vi "Skidpad.vi"() -> ()   [LabVIEW 2020]
uses:
  Control/SkidpadBestRecordIndicator.ctl
  Control/SkidpadCurrentRecordIndicator.ctl
  Control/SkidpadInternalVariable.ctl
  CommonControl/Flag.ctl
  Control/SkidpadInternalTimmer.ctl
  Control/SkidpadState.ctl
  <vilib>/DAQmx/write.llb/DAQmx Write (Analog DBL 1Chan 1Samp).vi
  <vilib>/DAQmx/read.llb/DAQmx Read (Analog DBL 1Chan 1Samp).vi
  <vilib>/DAQmx/create/channels.llb/DAQmx Create Channel (AO-Voltage-Basic).vi
  <vilib>/DAQmx/create/channels.llb/DAQmx Create Channel (AI-Voltage-Basic).vi
  <vilib>/Utility/file.llb/Read Delimited Spreadsheet (string).vi
  <vilib>/DAQmx/miscellaneous.llb/DAQmx Fill In Error Info.vi
  <vilib>/Utility/file.llb/Write Delimited Spreadsheet (string).vi
panel:
  out "Progress":string[][](table)
  in  "DNF":bool
  in  "DeviceName":tag
  in  "NextEntry":bool
  in  "Ready":bool
  in  "Retry":bool
  out "CurrentRecordIndicator":T1
  out "BestRecordIndicator":T2
  in  "ProgramStop":bool
  # "2023 KSAE Formula Skidpad Event"
  # "Team"
  # "Entry"
  # "Hit"
  # "University"
  # "Lap2 :"
  # "Lap4 :"
  # "Total :"
  # "Entry :"
  # "#1"
  # "#2"
  # "#3"
  # "#4"
  # "Univ. :"
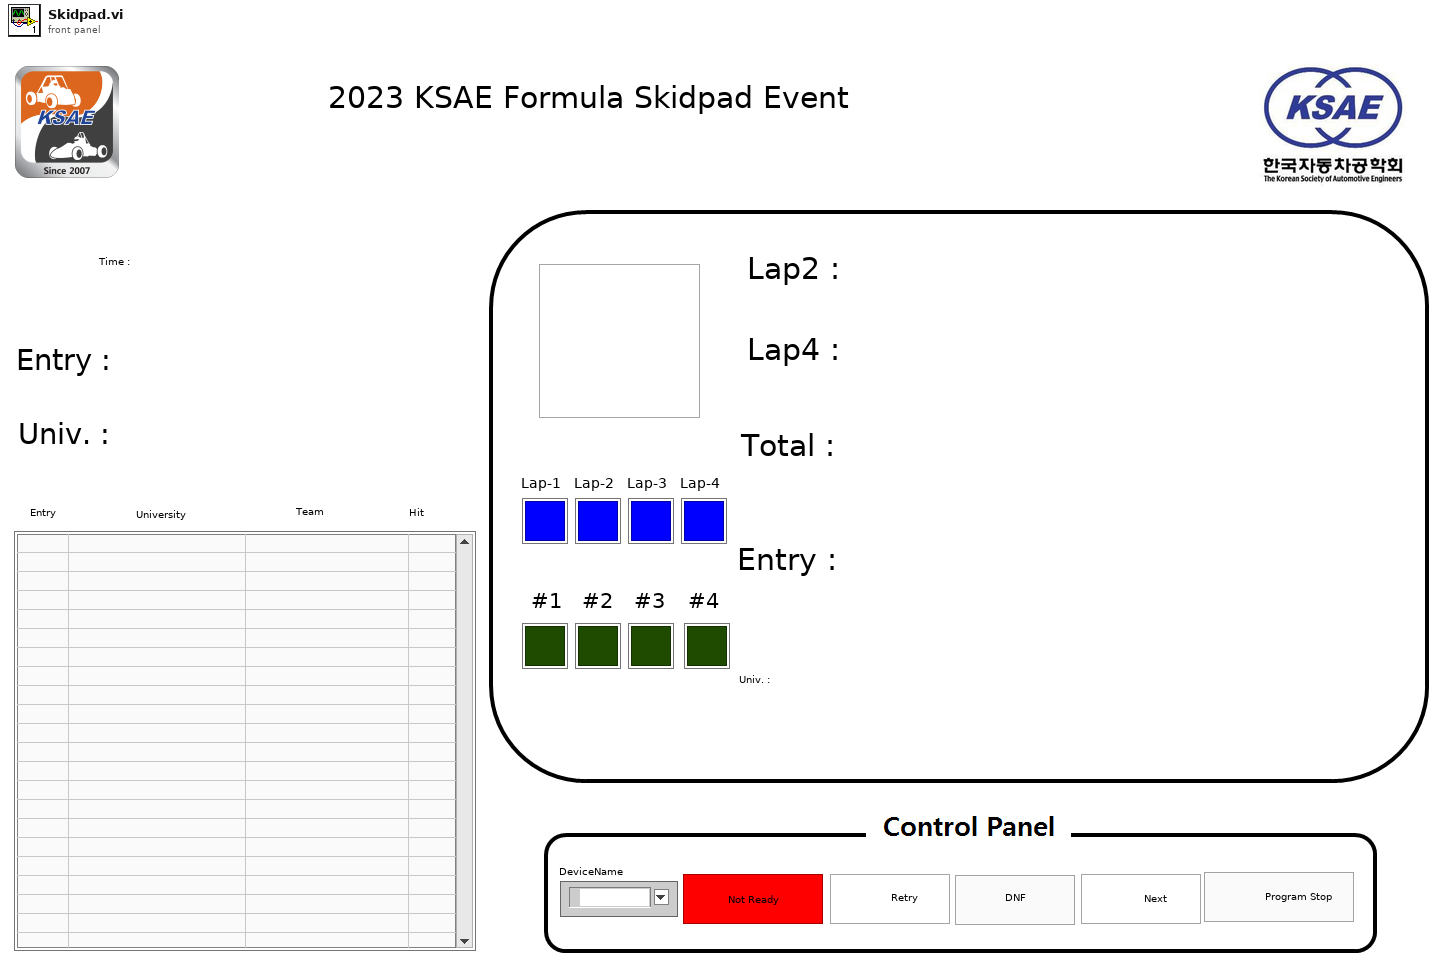
[diagram p1: front panel]
types:
  T1 = typedef "SkidpadCurrentRecordIndicator.ctl" = cluster{"Lab2":string, "Lab4":string, "TotalLabTime":string, "CurrentEntry":string, "CurrentSchool":string, "Flag":picture, "Message":string, "LapProgress":cluster{"Lap-1":bool, "Lap-2":bool, "Lap-3":bool, "Lap-4":bool}, "EventCount":cluster{"Attempt-1":bool, "Attempt-2":bool, "Attempt-3":bool, "Attempt-4":bool}}
  T2 = typedef "SkidpadBestRecordIndicator.ctl" = cluster{"BestTime":string, "BestEntry":string, "BestUniv":string}
  T3 = typedef "SkidpadInternalVariable.ctl" = cluster{"CurrentRecordIndicator":T1, "BestRecordIndicator":T2, "FlagData":T4, "InternalTimmer":T5, "StateValue":T6, "EventProgressData":string[][], "Ready":bool, "Retry":bool, "DNF":bool, "NextEntry":bool, "ProgramStop":bool}
  T4 = typedef "Flag.ctl" = cluster{"GreenFlag":picture, "BlueFlag":picture, "RedFlag":picture, "CheckFlag":picture}
  T5 = typedef "SkidpadInternalTimmer.ctl" = cluster{"1LapRefTime":i64, "1LapTime":i64, "2LapRefTime":i64, "2LapTime":i64, "3LapRefTime":i64, "3LapTime":i64, "4LapRefTime":i64, "4LapTime":i64, "TotalLabTime":i64}
  T6 = typedef "SkidpadState.ctl" = enum16{"Initial", "InputInfomation", "Ready", "1lap", "2lap", "3lap", "4lap", "FinshRunning", "LogRecord", "HardwareRelease", "WaittingforNext", "ProgramStop"}
  T7 = cluster{"Lap-1":bool, "Lap-2":bool, "Lap-3":bool, "Lap-4":bool}
  T8 = cluster{"CurrentEntry":string, "CurrentUniversity":string, "CurrentTeam":string}
  T9 = cluster{"Attempt-1":bool, "Attempt-2":bool, "Attempt-3":bool, "Attempt-4":bool}
  T10 = cluster{"Lab1":bool, "Lab2":bool, "Lab3":bool, "Lab4":bool}
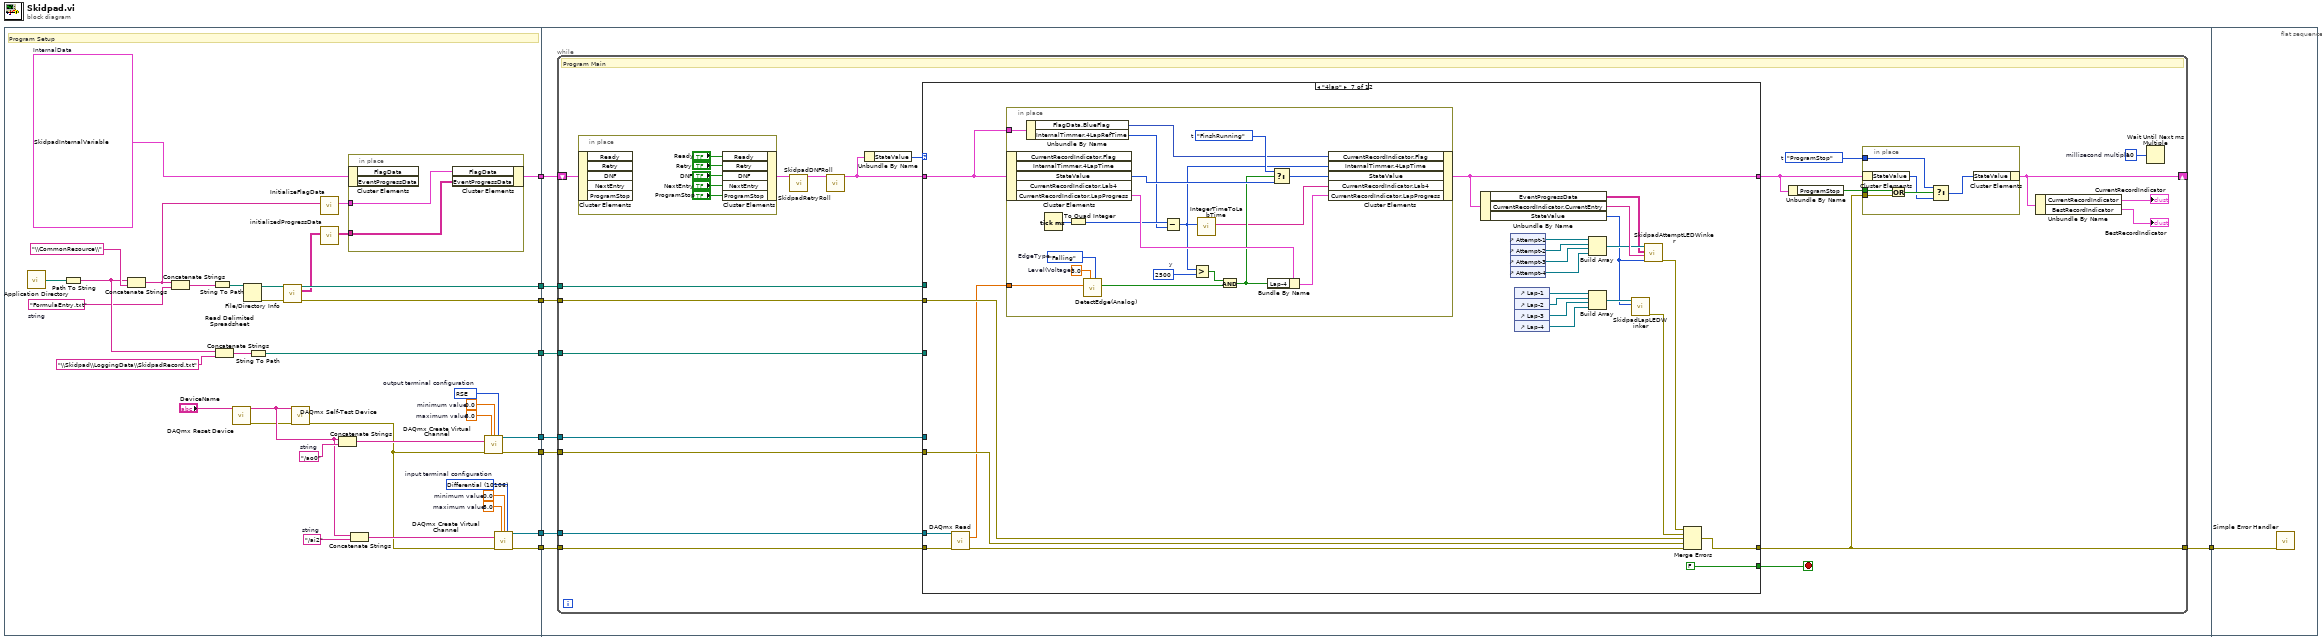
[diagram p0: block diagram]
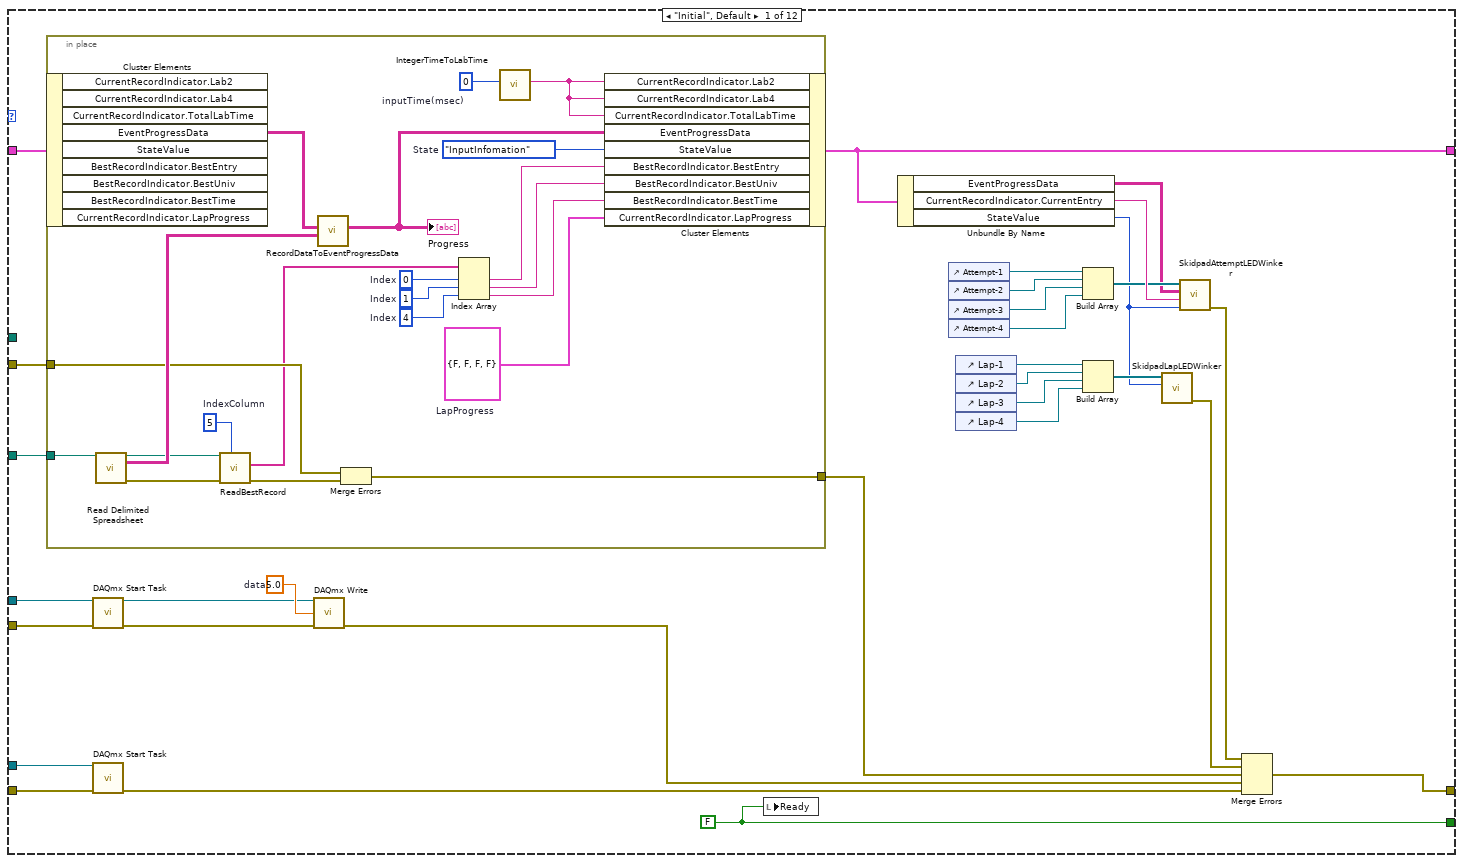
[diagram p2: hidden frame]
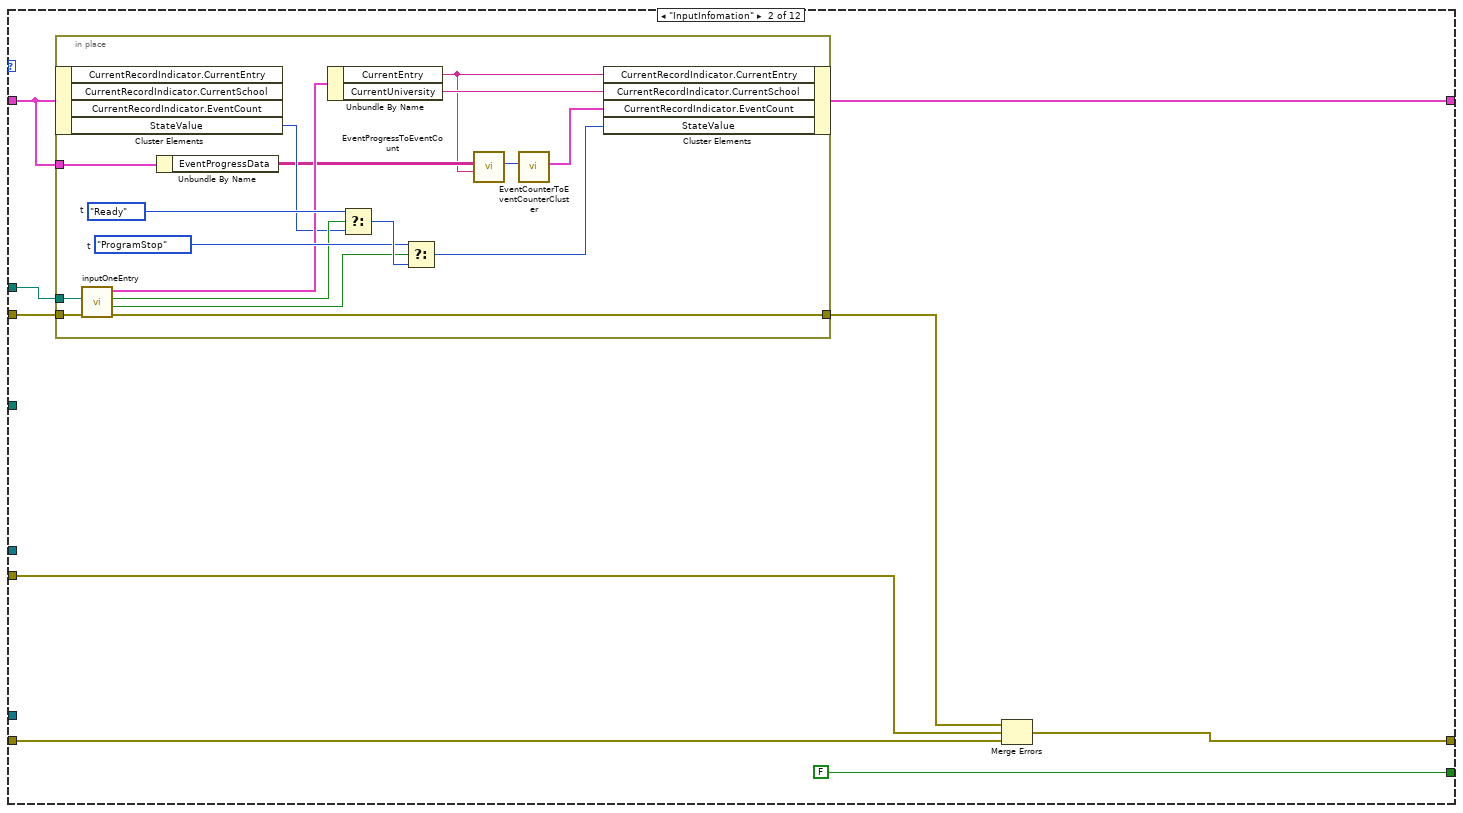
[diagram p3: hidden frame]
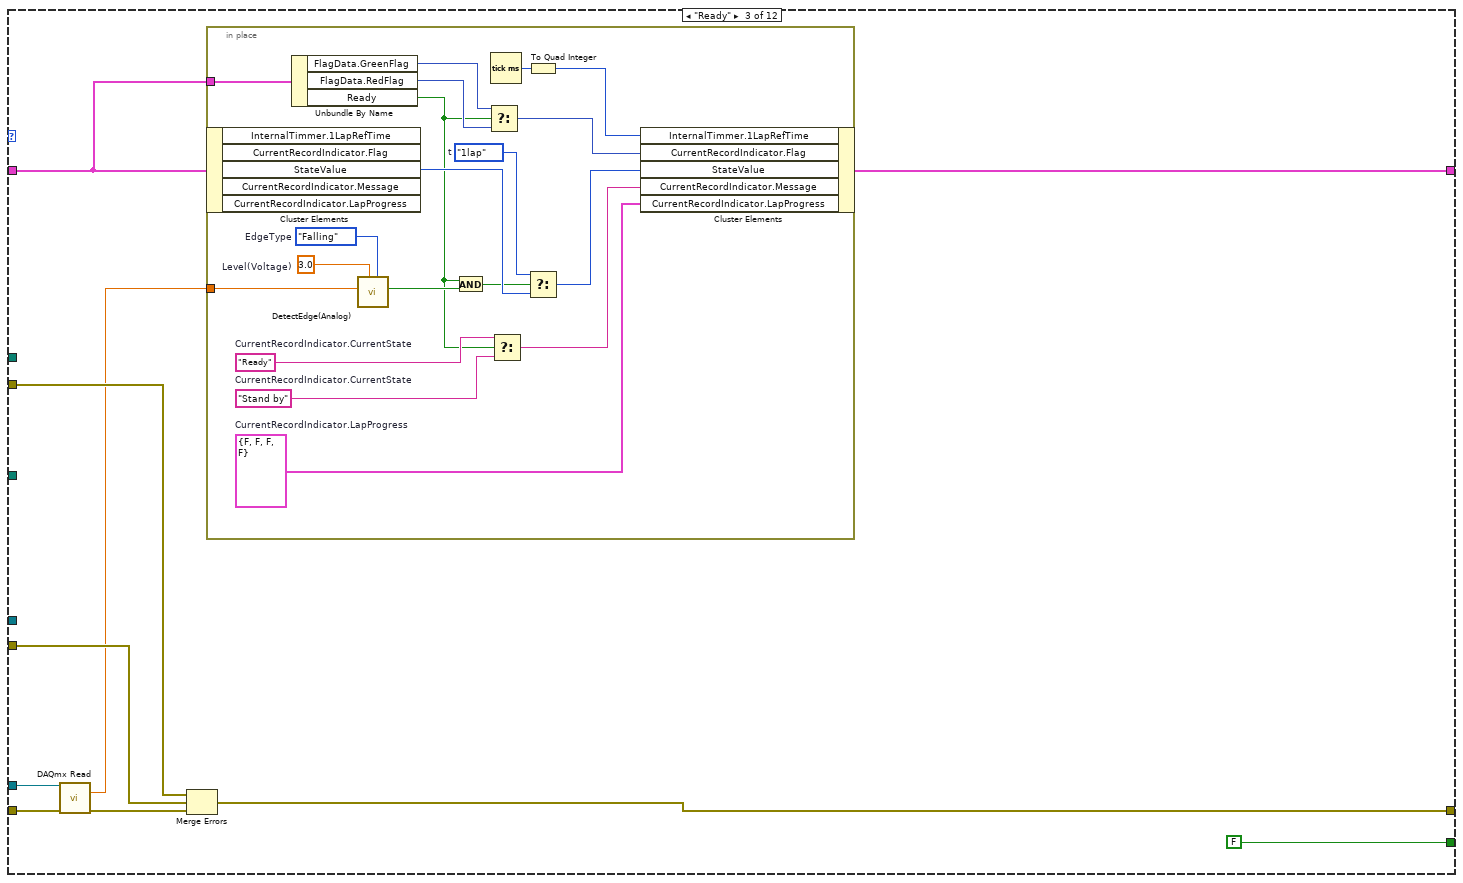
[diagram p4: hidden frame]
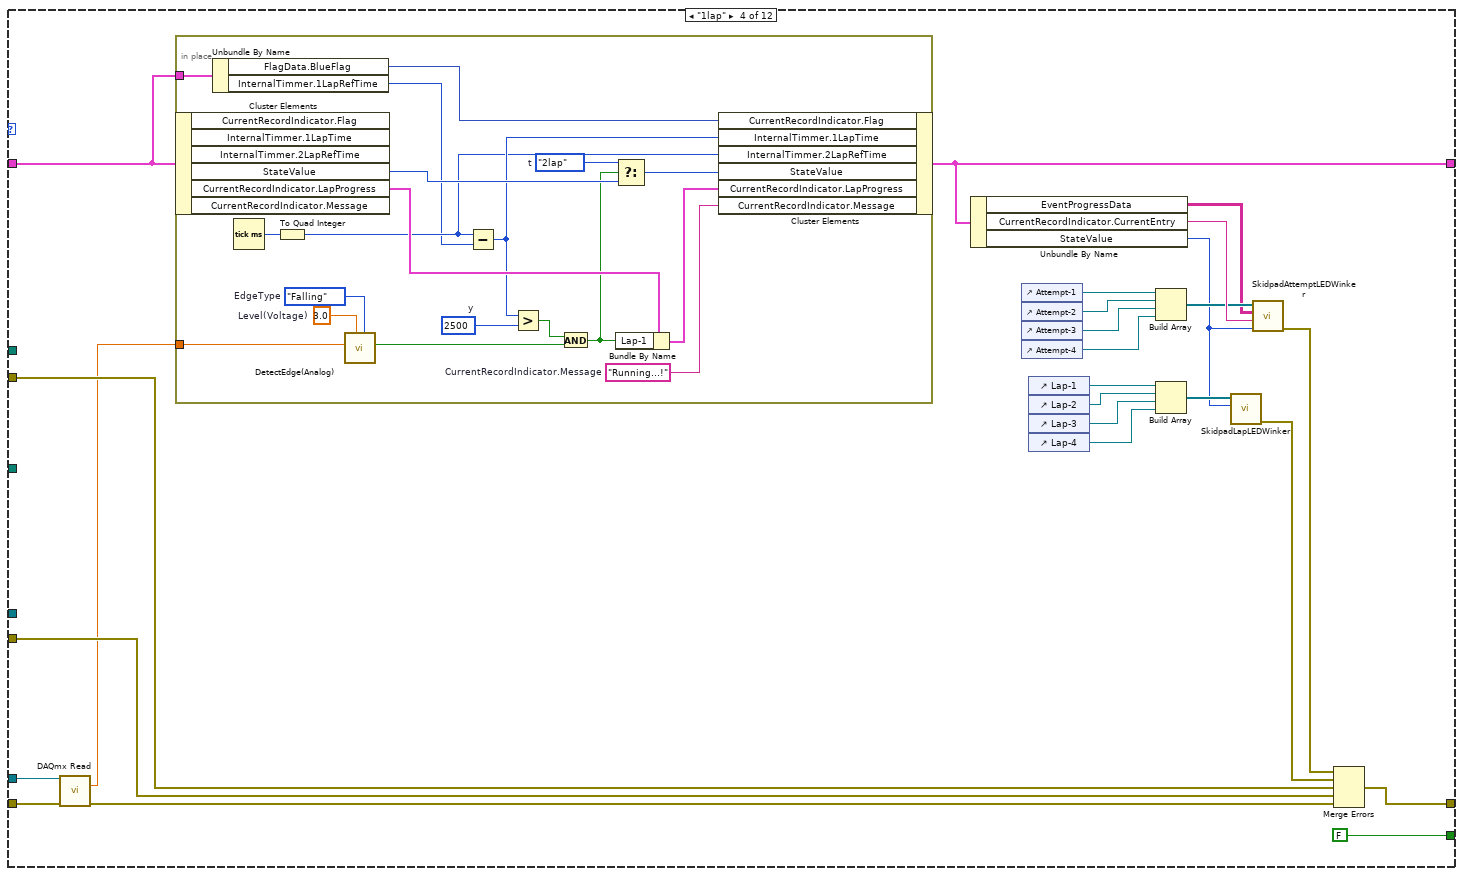
[diagram p5: hidden frame]
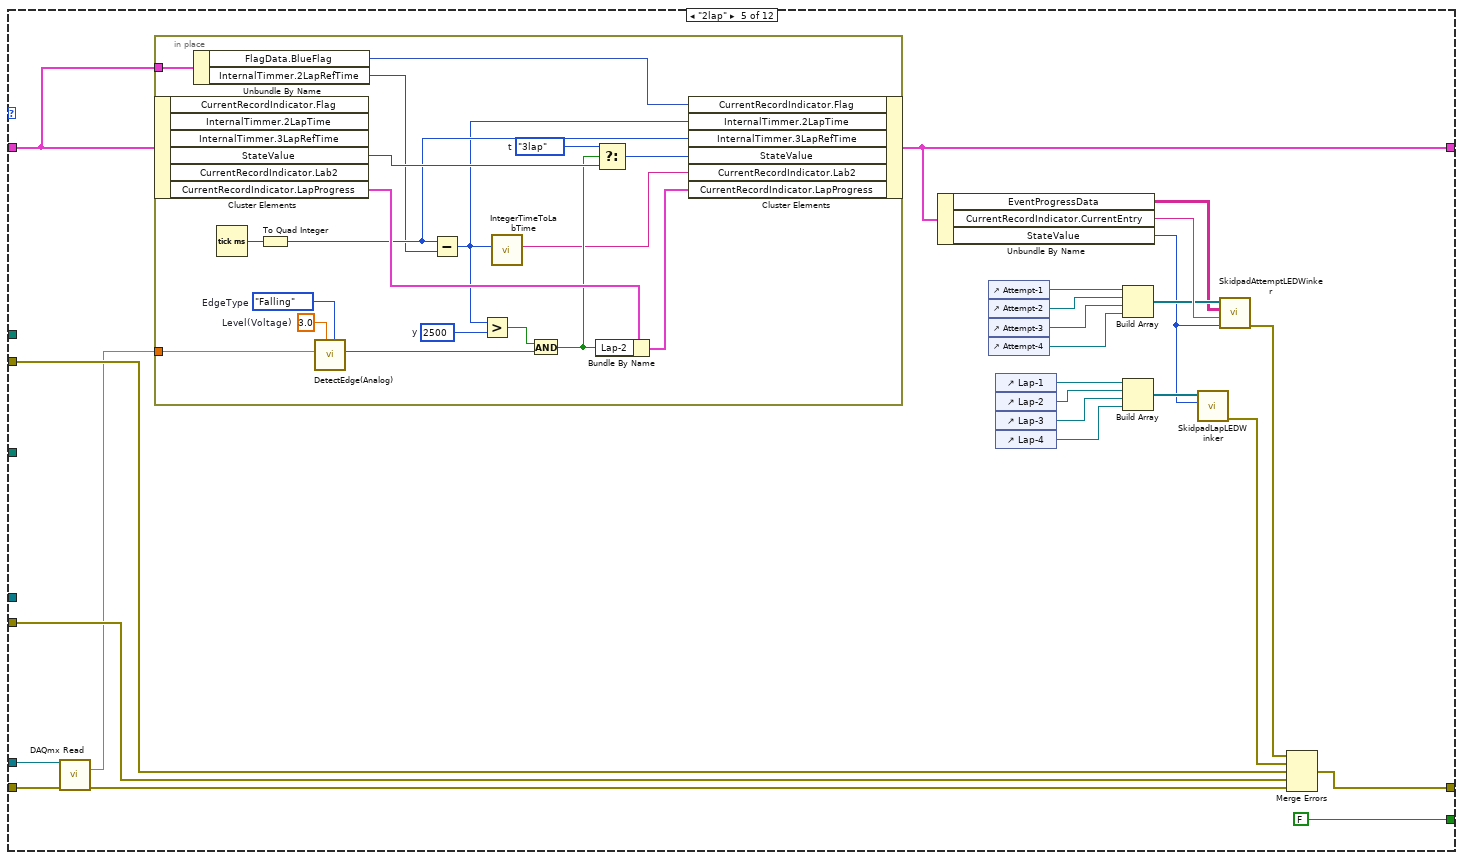
[diagram p6: hidden frame]
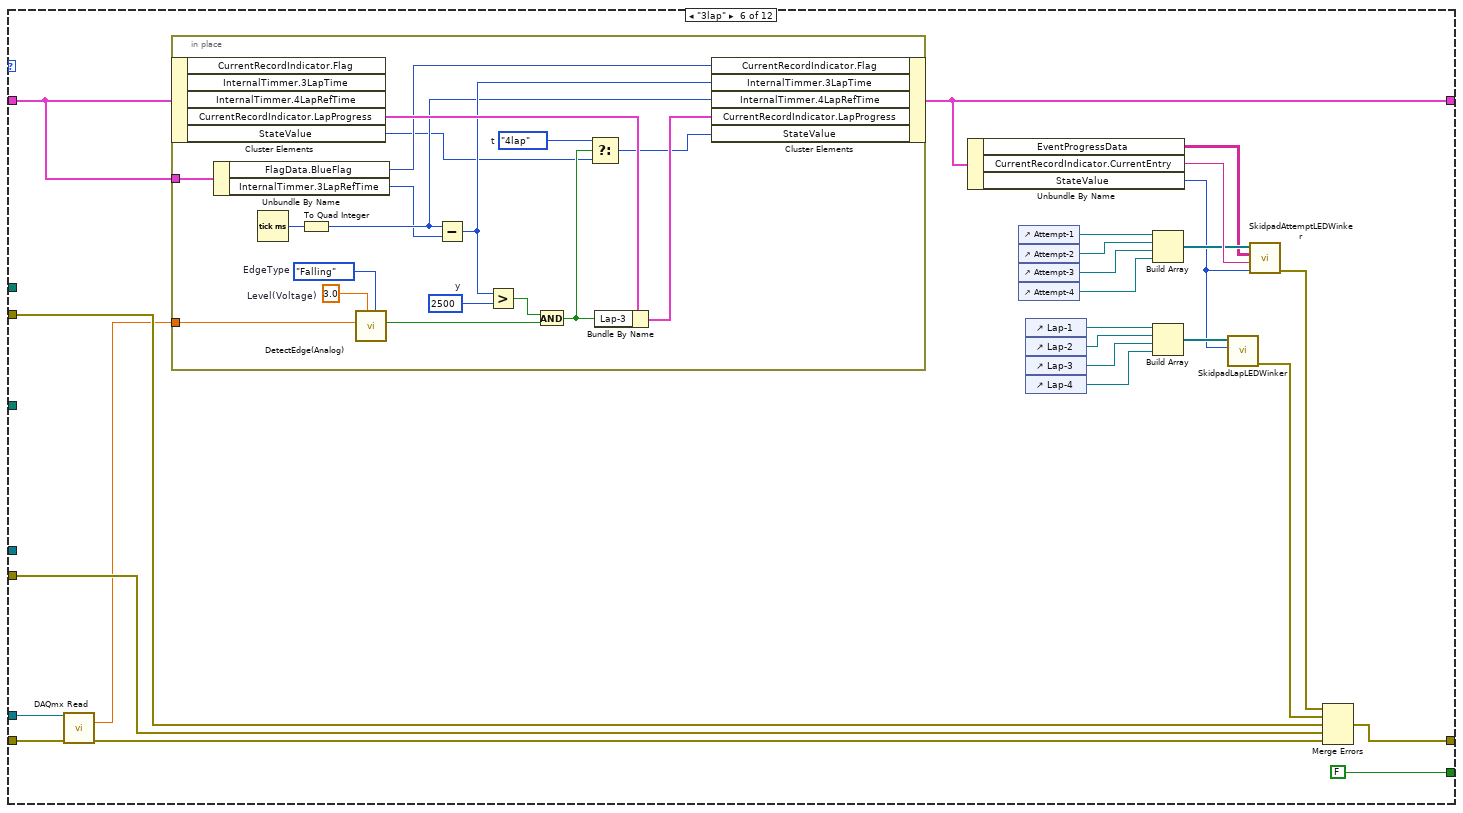
[diagram p7: hidden frame]
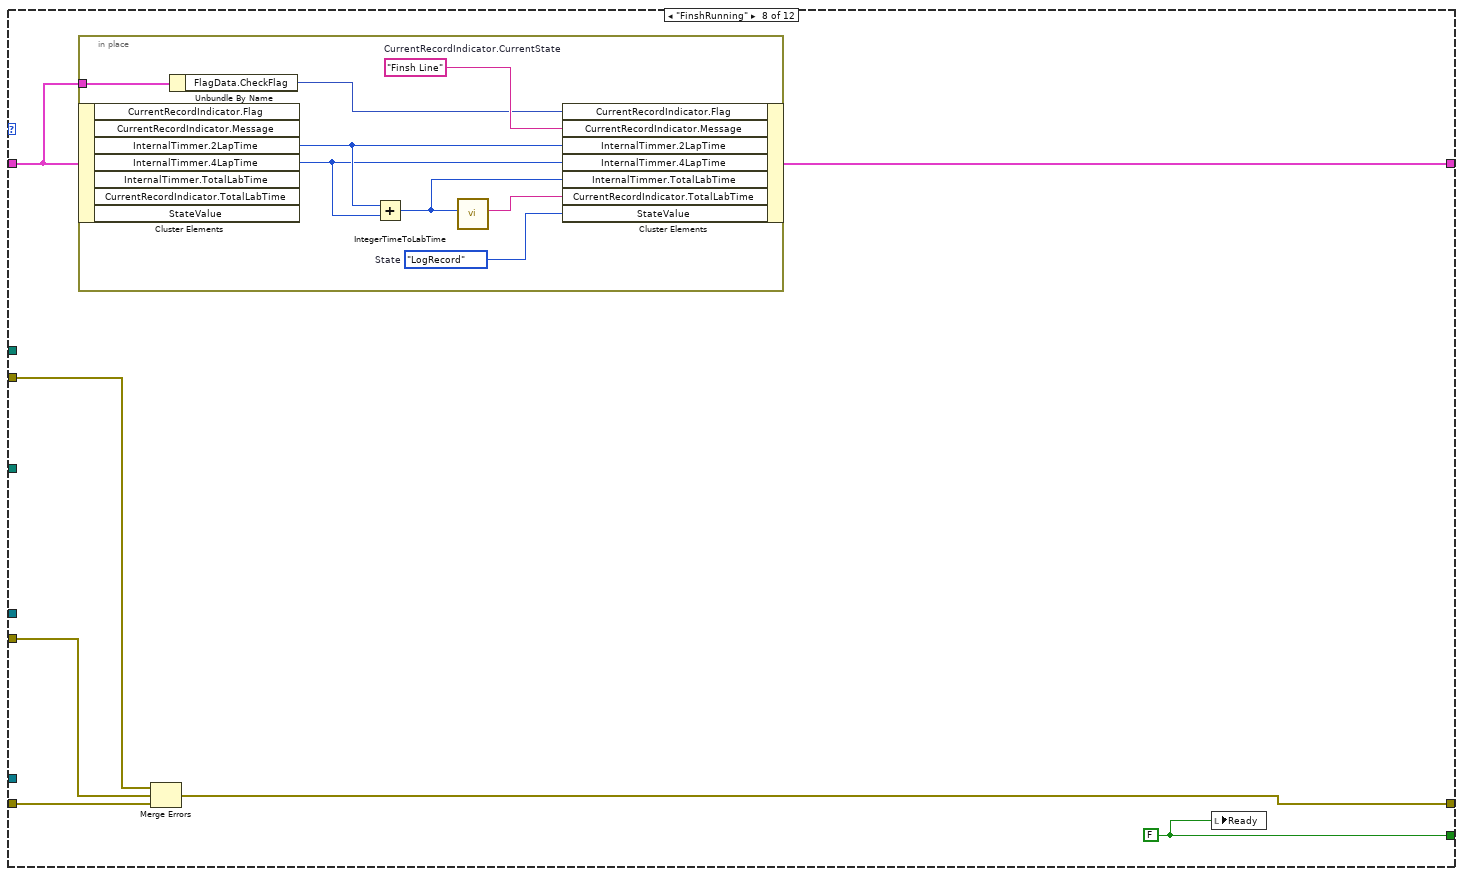
[diagram p8: hidden frame]
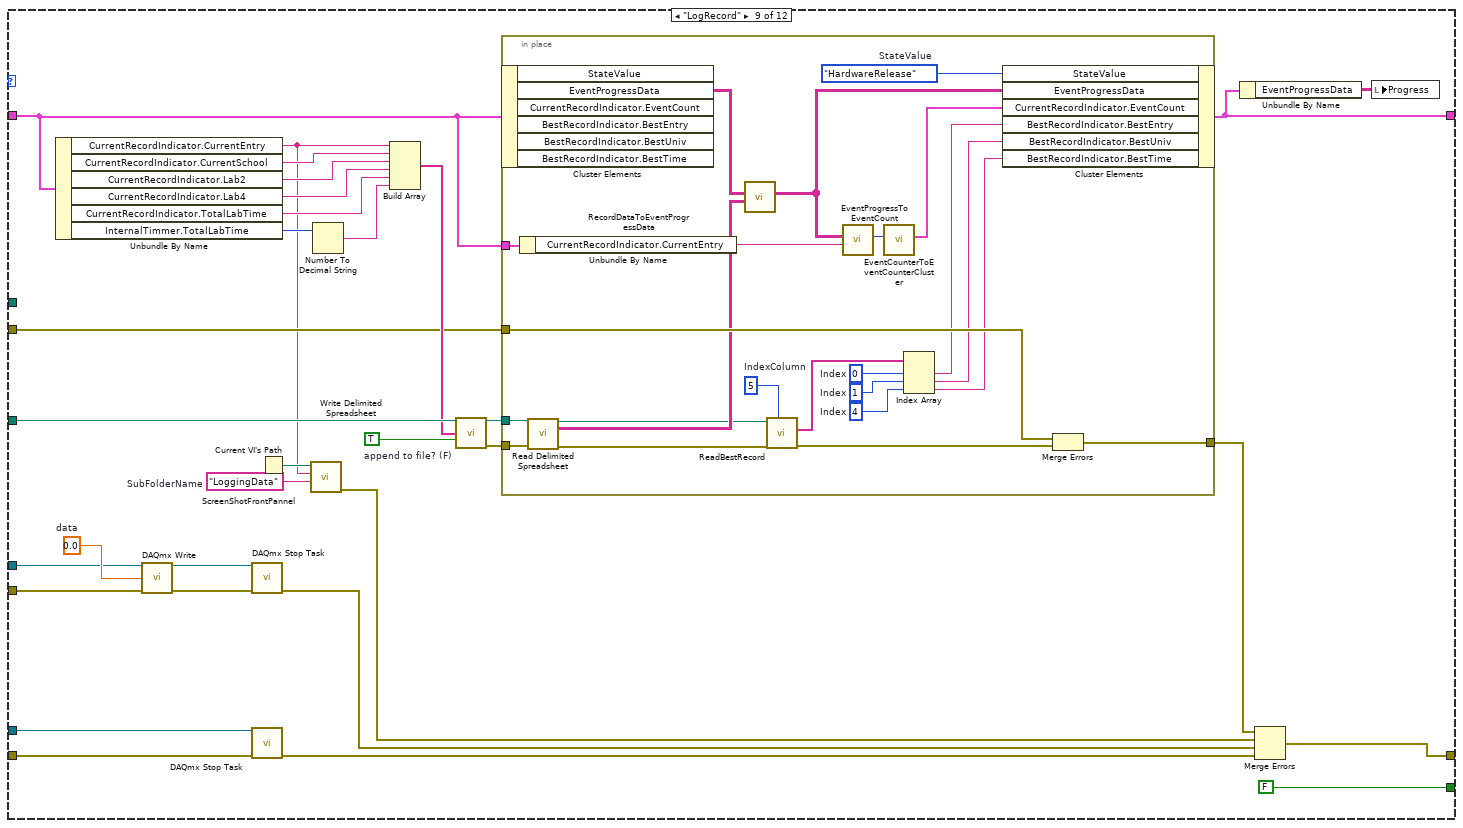
[diagram p9: hidden frame]
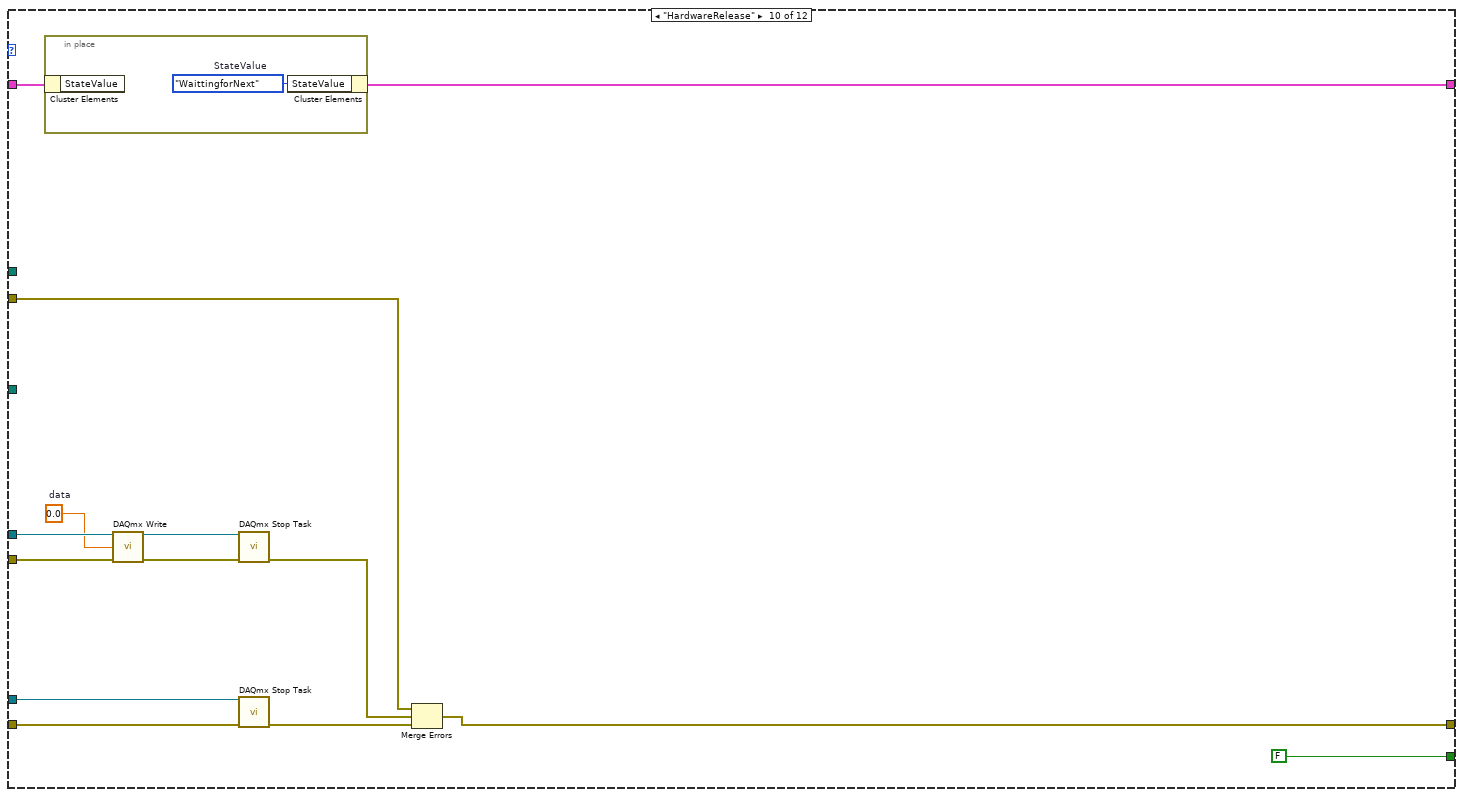
[diagram p10: hidden frame]
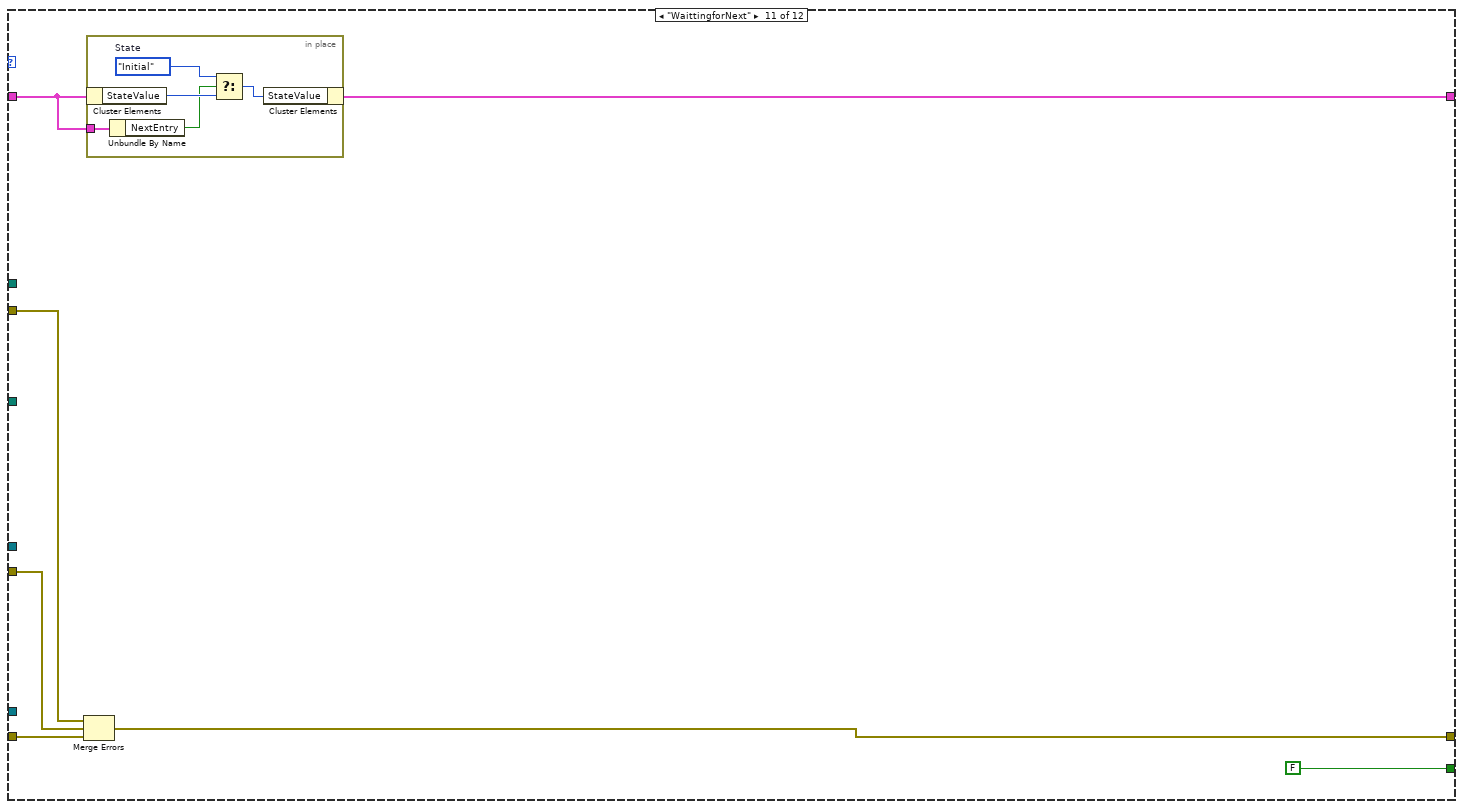
[diagram p11: hidden frame]
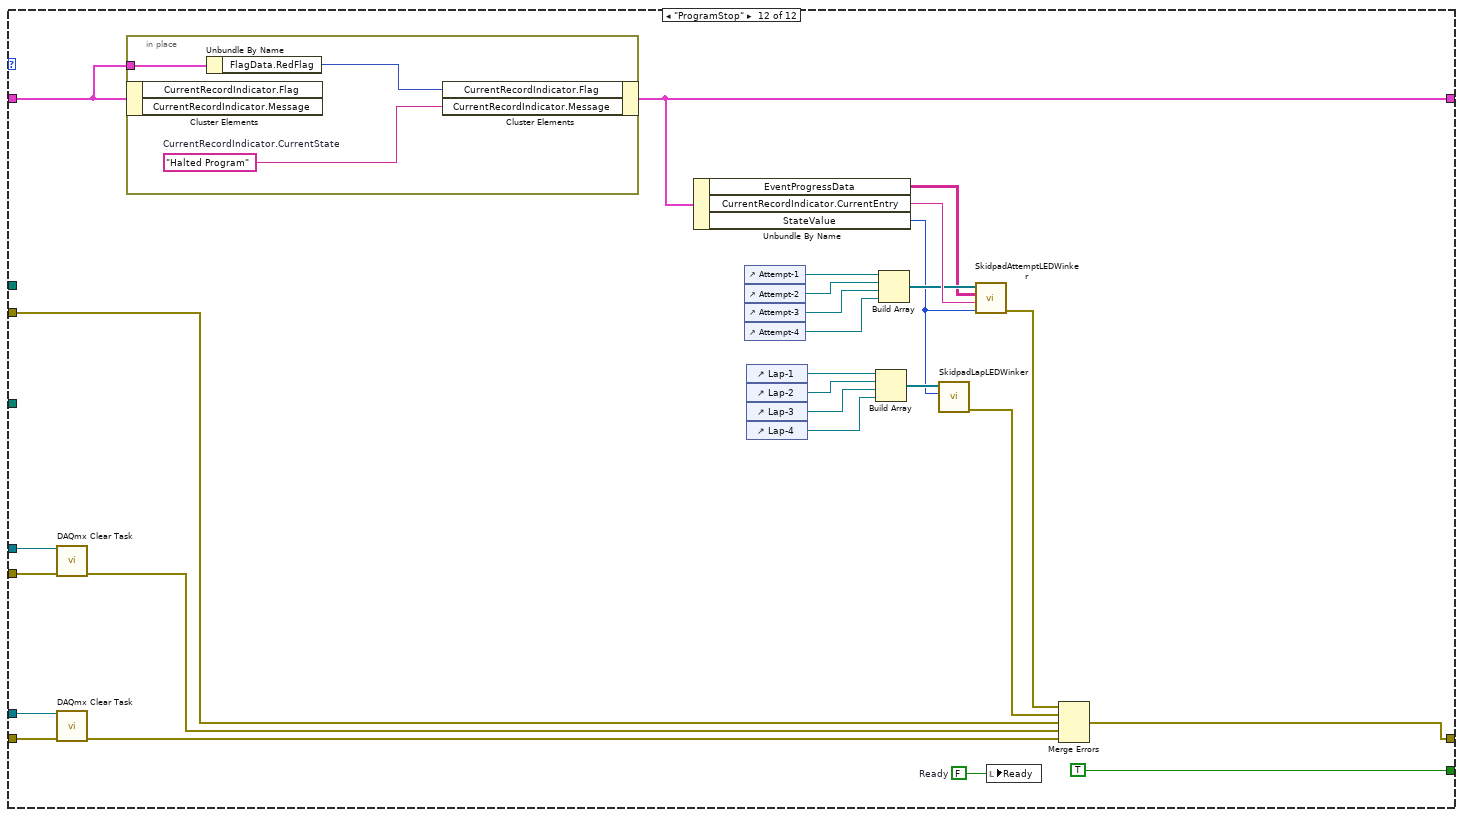
[diagram p12: hidden frame]
diagram:
  n1 = flat-sequence {
    tunnel: [w16] -> w9
    tunnel: [w44] -> w8
    tunnel: [w41] -> w7
    tunnel: [w23] -> w6
    tunnel: [w10] -> w5
    tunnel: [w19] -> w4
    tunnel: [w18] -> w3
    tunnel: [w14] -> w1
    tunnel: w9 -> [w56]
    tunnel: w8 -> [w52]
    tunnel: w7 -> [w53]
    tunnel: w6 -> [w55]
    tunnel: w5 -> [w54]
    tunnel: w4 -> [w51]
    tunnel: w3 -> [w50]
    tunnel: [w49] -> w2
    tunnel: w1 -> [w48]
    tunnel: w2 -> [w497]
    frame #0 {
      w11 = T3 {"CurrentRecordIndicator"={"Lab2"="", "Lab4"="", "TotalLabTime"="", "CurrentEntry"="", "CurrentSchool"="", "Flag"=bytes[0], "Message"="", "LapProgress"={"Lap-1"=FALSE, "Lap-2"=FALSE, "Lap-3"=FALSE, "Lap-4"=FALSE}, "EventCount"={"Attempt-1"=FALSE, "Attempt-2"=FALSE, "Attempt-3"=FALSE, "Attempt-4"=FALSE}}, "BestRecordIndicator"={"BestTime"="", "BestEntry"="", "BestUniv"=""}, "FlagData"={"GreenFlag"=bytes[0], "BlueFlag"=bytes[0], "RedFlag"=bytes[0], "CheckFlag"=bytes[0]}, "InternalTimmer"={"1LapRefTime"=0, "1LapTime"=0, "2LapRefTime"=0, "2LapTime"=0, "3LapRefTime"=0, "3LapTime"=0, "4LapRefTime"=0, "4LapTime"=0, "TotalLabTime"=0}, "StateValue"=enum."Initial", "EventProgressData"=[], "Ready"=FALSE, "Retry"=FALSE, "DNF"=FALSE, "NextEntry"=FALSE, "ProgramStop"=FALSE}  # InternalData
      w27 = "FormulaEntry.txt"  # string
      w36 = "/ai2"  # string
      w37 = "/ao0"  # string
      w38 = 10083 items=["Default"=-1, "RSE"=10083, "Differential"=10106, "Pseudodifferential"=12529]  # output terminal configuration
      w39 = 0.0  # minimum value
      w40 = 5.0  # maximum value
      w43 = 5.0  # maximum value
      w42 = 0.0  # minimum value
      w45 = 10106 items=["default"=-1, "RSE"=10083, "NRSE"=10078, "Differential"=10106, "Pseudodifferential"=12529]  # input terminal configuration
      # "Program Setup"
      n2 = call <vilib>:"Application Directory.vi"() -> ("Application Directory"=w33:path)
      n3 = Path To String(path=w33) -> (string=w29:string)
      n4 = Concatenate Strings "Concatenate Strings"(w29, "\\CommonResource\\") -> (w12:string)
      n5 = Concatenate Strings "Concatenate Strings"(w12, w27) -> (w28:string)
      n6 = String To Path(string=w28) -> (path=w26:path)
      n7 = Concatenate Strings "Concatenate Strings"(w29, "\\Skidpad\\LoggingData\\SkidpadRecord.txt") -> (w31:string)
      n8 = call <vilib>:"DAQmx Reset Device.vi"("device in"="DeviceName") -> ("error out"=w21:errorcluster)  [unwired: 14 in]
      n9 = File/Directory Info(path=w26) -> (path out=w25:path, error out=w24:errorcluster)  [unwired: 1 in, 5 out]
      n10 = String To Path(string=w31) -> (path=w10:path)
      n11 = call-poly <vilib>:"Read Delimited Spreadsheet.vi"("file path (dialog if empty)"=w25, "error in (no error)"=w24) -> ("new file path (Not A Path if cancelled)"=w23:path, "all rows"=w17:string[][], "error out"=w14:errorcluster)  [unwired: 8 in, 3 out]
      n12 = call <vilib>:"DAQmx Self-Test Device.vi"("device in"="DeviceName", "error in"=w21) -> ("error out"=w20:errorcluster)  [unwired: 13 in]
      n13 = call "initializedProgressData.vi"("inputEntry"=w17) -> ("outputProgressData"=w15:string[][])  [unwired: 10 in]
      n14 = call "InitializeFlagData.vi"("inputPath"=w12) -> ("outputFlagData"=w13:T4)  [unwired: 9 in, 1 out]
      n15 = Concatenate Strings "Concatenate Strings"("DeviceName", w37) -> (w34:string)
      n16 = in-place {
        in-place-border: w15 -> [w46]
        in-place-border: w13 -> [w47]
        n17 = in-place-cluster #1(w11) -> ()  [unwired: 2 out]
        n18 = in-place-cluster #1("FlagData"=w47, "EventProgressData"=w46) -> (w16:T3)
      }
      n19 = Concatenate Strings "Concatenate Strings"("DeviceName", w36) -> (w35:string)
      n20 = call-poly <vilib>:"DAQmx Create Virtual Channel.vi"("maximum value"=w40, "minimum value"=w39, "output terminal configuration"=w38, "physical channels"=w34, "error in"=w20) -> ("task out"=w41:refnum<k21>, "error out"=w19:errorcluster)  [unwired: 9 in]
      n21 = call-poly <vilib>:"DAQmx Create Virtual Channel.vi"("maximum value"=w43, "minimum value"=w42, "input terminal configuration"=w45, "physical channels"=w35, "error in"=w20) -> ("task out"=w44:refnum<k21>, "error out"=w18:errorcluster)  [unwired: 9 in]
    }
    frame #1 {
      n22 = while {
        tunnel: w52 -> [w77]
        shift-right: [w73] -> _
        shift-left: w56 -> [w64]
        tunnel: w53 -> [w71]
        tunnel: w55 -> [w70]
        tunnel: w54 -> [w69]
        tunnel: w51 -> [w68]
        tunnel: w50 -> [w67]
        tunnel: [w58] -> w49
        tunnel: w48 -> [w65]
        stop <- w72 stop-if-true
        w57 = SkidpadState."ProgramStop"  # t
        w66 = u32 10  # millisecond multiple
        # "Program Main"
        n23 = in-place {
          n24 = in-place-cluster #2(w64) -> ()  [unwired: 5 out]
          n25 = in-place-cluster #2("Ready"="Ready", "Retry"="Retry", "DNF"="DNF", "NextEntry"="NextEntry", "ProgramStop"="ProgramStop") -> (w62:T3)
        }
        n26 = call "SkidpadDNFRoll.vi"("inputInternalData"=w62) -> ("outputInternalData"=w60:T3)  [unwired: 10 in]
        n27 = call "SkidpadRetryRoll.vi"("InternalData"=w60) -> ("InternalData 2"=w59:T3)  [unwired: 10 in]
        n28 = Unbundle By Name(w59) -> ("StateValue"=w76:T6)
        n29 = case shown="\"4lap\"" w76 {
          tunnel: w77 -> [w109 _ w170 w214 w258 w302 w345 _ w400 w442 _ w487]
          tunnel: w67 -> [w108 w136 w169 w213 w257 w301 w344 w367 w398 w441 w451 w482]
          tunnel: w59 -> [w113 w137 w165 w210 w254 w298 w341 w366 w380 w447 w449 w478]
          tunnel: [w84 w139 w168 w193 w237 w281 w324 w371 w388 w435 w454 w463] -> w61
          tunnel: [w83 FALSE FALSE FALSE FALSE FALSE FALSE w365 FALSE FALSE FALSE TRUE] -> w72
          tunnel: [w107 w143 w164 w209 w253 w297 w340 w370 w397 w437 w453 w484] -> w58
          tunnel: w69 -> [w112 _ _ _ _ _ _ _ w394 _ _ _]
          tunnel: w71 -> [w111 _ _ _ _ _ _ _ w401 w446 _ w485]
          tunnel: w70 -> [_ w140 _ _ _ _ _ _ _ _ _ _]
          tunnel: w68 -> [w110 w135 w163 w208 w252 w296 w339 w368 w399 w445 w452 w481]
          tunnel: w65 -> [w100 w138 w162 w207 w251 w295 w338 w369 w389 w438 w450 w477]
          frame "Initial", Default {
            w104 = 5.0  # data
            w83 = FALSE
            n30 = in-place {
              in-place-border: w112 -> [w133]
              in-place-border: [w128] -> w105
              in-place-border: w100 -> [w127]
              w114 = T7 {"Lap-1"=FALSE, "Lap-2"=FALSE, "Lap-3"=FALSE, "Lap-4"=FALSE}  # LapProgress
              w122 = 5  # IndexColumn
              w123 = 4  # Index
              w124 = 1  # Index
              w125 = 0  # Index
              w134 = i64 0  # inputTime(msec)
              w130 = SkidpadState."InputInfomation"  # State
              n31 = in-place-cluster #3(w113) -> ("EventProgressData"=w131:string[][])  [unwired: 8 out]
              n32 = call-poly <vilib>:"Read Delimited Spreadsheet.vi"("file path (dialog if empty)"=w133) -> ("new file path (Not A Path if cancelled)"=w121:path, "all rows"=w132:string[][], "error out"=w120:errorcluster)  [unwired: 9 in, 3 out]
              n33 = call "ReadBestRecord.vi"("IndexColumn"=w122, "ErrorInput"=w120, "FilepathInput"=w121) -> ("ErrorOutput"=w119:errorcluster, "Data"=w126:string[])  [unwired: 6 in, 1 out]
              n34 = call "RecordDataToEventProgressData.vi"("RecordData"=w132, "inputEventProgressData"=w131) -> ("outputEventProgressData"=w129:string[][])  [unwired: 9 in]
              "Progress" <- w129
              n35 = Merge Errors "Merge Errors"(w127, w119) -> (w128:errorcluster)
              n36 = Index Array "Index Array"(array=w126, index #1=w125, index #2=w124, index #3=w123) -> (element #1=w117:string, element #2=w116:string, element #3=w115:string)
              n37 = call "IntegerTimeToLabTime.vi"("inputTime(msec)"=w134) -> ("outputTime(mm-ss-sss)"=w118:string)  [unwired: 10 in]
              n38 = in-place-cluster #3("CurrentRecordIndicator.Lab2"=w118, "CurrentRecordIndicator.Lab4"=w118, "CurrentRecordIndicator.TotalLabTime"=w118, "EventProgressData"=w129, "StateValue"=w130, "BestRecordIndicator.BestEntry"=w117, "BestRecordIndicator.BestUniv"=w116, "BestRecordIndicator.BestTime"=w115, "CurrentRecordIndicator.LapProgress"=w114) -> (w84:T3)
            }
            n39 = call <vilib>:"DAQmx Start Task.vi"("task/channels in"=w111, "error in"=w110) -> ("task out"=w102:refnum<k21>, "error out"=w103:errorcluster)  [unwired: 12 in]
            n40 = call <vilib>:"DAQmx Start Task.vi"("task/channels in"=w109, "error in"=w108) -> ("error out"=w106:errorcluster)  [unwired: 12 in, 1 out]
            n41 = call-poly <vilib>:"DAQmx Write.vi"("task/channels in"=w102, "data"=w104, "error in"=w103) -> ("error out"=w101:errorcluster)  [unwired: 10 in, 2 out]
            n42 = local write "Ready"(w83) -> ()
            n43 = Unbundle By Name(w84) -> ("EventProgressData"=w86:string[][], "CurrentRecordIndicator.CurrentEntry"=w93:string, "StateValue"=w87:T6)
            n44 = control-ref of="Attempt-1"() -> (w88:refnum<vi>)
            n45 = control-ref of="Attempt-2"() -> (w89:refnum<vi>)
            n46 = control-ref of="Attempt-3"() -> (w90:refnum<vi>)
            n47 = control-ref of="Attempt-4"() -> (w91:refnum<vi>)
            n48 = control-ref of="Lap-1"() -> (w95:refnum<vi>)
            n49 = control-ref of="Lap-2"() -> (w96:refnum<vi>)
            n50 = control-ref of="Lap-3"() -> (w97:refnum<vi>)
            n51 = control-ref of="Lap-4"() -> (w98:refnum<vi>)
            n52 = Build Array "Build Array"(w88, w89, w90, w91) -> (w92:refnum<vi>[])
            n53 = Build Array "Build Array"(w95, w96, w97, w98) -> (w99:refnum<vi>[])
            n54 = call "SkidpadLapLEDWinker.vi"("StateValue"=w87, "inputRefOfLED"=w99) -> ("outputError"=w94:errorcluster)  [unwired: 9 in]
            n55 = call "SkidpadAttemptLEDWinker.vi"("StateValue"=w87, "CurrentEntry"=w93, "EventProgressDataInput"=w86, "inputRefOfLED"=w92) -> ("outputError"=w85:errorcluster)  [unwired: 7 in]
            n56 = Merge Errors "Merge Errors"(w85, w94, w105, w101, w106) -> (w107:errorcluster)
          }
          frame "InputInfomation" {
            n57 = in-place {
              in-place-border: [w157] -> w142
              in-place-border: w140 -> [w155]
              in-place-border: w138 -> [w154]
              in-place-border: w137 -> [w149]
              w158 = SkidpadState."ProgramStop"  # t
              w160 = SkidpadState."Ready"  # t
              n58 = in-place-cluster #4(w137) -> ("StateValue"=w150:T6)  [unwired: 3 out]
              n59 = call "inputOneEntry.vi"("inputError"=w154, "file path (dialog if empty)"=w155) -> ("outputError"=w157:errorcluster, "StopButtonOutput"=w151:bool, "OKButtonOutput"=w152:bool, "CurrentData"=w153:T8)  [unwired: 6 in]
              n60 = Unbundle By Name(w149) -> ("EventProgressData"=w148:string[][])
              n61 = Unbundle By Name(w153) -> ("CurrentEntry"=w147:string, "CurrentUniversity"=w156:string)
              n62 = Select(t=w160, s=w152, f=w150) -> (s? t:f=w159:T6)
              n63 = Select(t=w158, s=w151, f=w159) -> (s? t:f=w145:T6)
              n64 = call "EventProgressToEventCount.vi"("CurrentEntry"=w147, "EventProgressDataInput"=w148) -> ("EventCount"=w146:i32)  [unwired: 9 in]
              n65 = call "EventCounterToEventCounterCluster.vi"("EventCount"=w146) -> ("CurrentRecordIndicator.EventCount"=w144:T9)  [unwired: 10 in]
              n66 = in-place-cluster #4("CurrentRecordIndicator.CurrentEntry"=w147, "CurrentRecordIndicator.CurrentSchool"=w156, "CurrentRecordIndicator.EventCount"=w144, "StateValue"=w145) -> (w139:T3)
            }
            n67 = Merge Errors "Merge Errors"(w142, w135, w136) -> (w143:errorcluster)
          }
          frame "Ready" {
            n68 = call-poly <vilib>:"DAQmx Read.vi"("task/channels in"=w170, "error in"=w169) -> ("data"=w161:dbl, "error out"=w167:errorcluster)  [unwired: 11 in, 1 out]
            n69 = Merge Errors "Merge Errors"(w162, w163, w167) -> (w164:errorcluster)
            n70 = in-place {
              in-place-border: w161 -> [w185]
              in-place-border: w165 -> [w176]
              w171 = enum16{"Rising", "Falling"}."Falling"  # EdgeType
              w178 = T10 {"Lab1"=FALSE, "Lab2"=FALSE, "Lab3"=FALSE, "Lab4"=FALSE}  # CurrentRecordIndicator.LapProgress
              w179 = "Stand by"  # CurrentRecordIndicator.CurrentState
              w182 = 3.0  # Level(Voltage)
              w180 = "Ready"  # CurrentRecordIndicator.CurrentState
              w187 = SkidpadState."1lap"  # t
              n71 = in-place-cluster #5(w165) -> ("StateValue"=w189:T6)  [unwired: 4 out]
              n72 = Unbundle By Name(w176) -> ("FlagData.GreenFlag"=w174:picture, "FlagData.RedFlag"=w175:picture, "Ready"=w172:bool)
              n73 = call "DetectEdge(Analog).vi"("EdgeType"=w171, "Level(Voltage)"=w182, "Voltage"=w185) -> ("DetectedEdge"=w186:bool)  [unwired: 8 in]
              n74 = And(x=w172, y=w186) -> (x .and. y?=w184:bool)
              n75 = Select(t=w174, s=w172, f=w175) -> (s? t:f=w183:picture)
              n76 = Tick Count (ms)() -> (millisecond timer value=w177:u32)
              n77 = Select(t=w180, s=w172, f=w179) -> (s? t:f=w181:string)
              n78 = To Quad Integer(1:w177) -> (0:w173:i64)
              n79 = Select(t=w187, s=w184, f=w189) -> (s? t:f=w188:T6)
              n80 = in-place-cluster #5("InternalTimmer.1LapRefTime"=w173, "CurrentRecordIndicator.Flag"=w183, "StateValue"=w188, "CurrentRecordIndicator.Message"=w181, "CurrentRecordIndicator.LapProgress"=w178) -> (w168:T3)
            }
          }
          frame "1lap" {
            n81 = call-poly <vilib>:"DAQmx Read.vi"("task/channels in"=w214, "error in"=w213) -> ("data"=w190:dbl, "error out"=w211:errorcluster)  [unwired: 11 in, 1 out]
            n82 = in-place {
              in-place-border: w190 -> [w231]
              in-place-border: w210 -> [w219]
              w215 = "Running...!"  # CurrentRecordIndicator.Message
              w216 = enum16{"Rising", "Falling"}."Falling"  # EdgeType
              w224 = i64 2500  # y
              w230 = 3.0  # Level(Voltage)
              w232 = SkidpadState."2lap"  # t
              n83 = in-place-cluster #6(w210) -> ("StateValue"=w233:T6, "CurrentRecordIndicator.LapProgress"=w229:T7)  [unwired: 4 out]
              n84 = Unbundle By Name(w219) -> ("FlagData.BlueFlag"=w218:picture, "InternalTimmer.1LapRefTime"=w217:i64)
              n85 = Tick Count (ms)() -> (millisecond timer value=w222:u32)
              n86 = To Quad Integer(1:w222) -> (0:w221:i64)
              n87 = call "DetectEdge(Analog).vi"("EdgeType"=w216, "Level(Voltage)"=w230, "Voltage"=w231) -> ("DetectedEdge"=w227:bool)  [unwired: 8 in]
              n88 = Subtract(x=w221, y=w217) -> (x-y=w225:i64)
              n89 = Greater?(x=w225, y=w224) -> (0:w223:bool)
              n90 = And(x=w223, y=w227) -> (x .and. y?=w226:bool)
              n91 = Select(t=w232, s=w226, f=w233) -> (s? t:f=w220:T6)
              n92 = Bundle By Name(cluster=w229, "Lap-1"=w226) -> (w228:T7)
              n93 = in-place-cluster #6("CurrentRecordIndicator.Flag"=w218, "InternalTimmer.1LapTime"=w225, "InternalTimmer.2LapRefTime"=w221, "StateValue"=w220, "CurrentRecordIndicator.LapProgress"=w228, "CurrentRecordIndicator.Message"=w215) -> (w193:T3)
            }
            n94 = Unbundle By Name(w193) -> ("EventProgressData"=w194:string[][], "CurrentRecordIndicator.CurrentEntry"=w201:string, "StateValue"=w195:T6)
            n95 = control-ref of="Attempt-1"() -> (w196:refnum<vi>)
            n96 = control-ref of="Attempt-2"() -> (w197:refnum<vi>)
            n97 = control-ref of="Attempt-3"() -> (w198:refnum<vi>)
            n98 = control-ref of="Attempt-4"() -> (w199:refnum<vi>)
            n99 = control-ref of="Lap-1"() -> (w202:refnum<vi>)
            n100 = control-ref of="Lap-2"() -> (w203:refnum<vi>)
            n101 = control-ref of="Lap-3"() -> (w204:refnum<vi>)
            n102 = control-ref of="Lap-4"() -> (w205:refnum<vi>)
            n103 = Build Array "Build Array"(w196, w197, w198, w199) -> (w200:refnum<vi>[])
            n104 = Build Array "Build Array"(w202, w203, w204, w205) -> (w206:refnum<vi>[])
            n105 = call "SkidpadLapLEDWinker.vi"("StateValue"=w195, "inputRefOfLED"=w206) -> ("outputError"=w191:errorcluster)  [unwired: 9 in]
            n106 = call "SkidpadAttemptLEDWinker.vi"("StateValue"=w195, "CurrentEntry"=w201, "EventProgressDataInput"=w194, "inputRefOfLED"=w200) -> ("outputError"=w192:errorcluster)  [unwired: 7 in]
            n107 = Merge Errors "Merge Errors"(w192, w191, w207, w208, w211) -> (w209:errorcluster)
          }
          frame "2lap" {
            n108 = call-poly <vilib>:"DAQmx Read.vi"("task/channels in"=w258, "error in"=w257) -> ("data"=w234:dbl, "error out"=w255:errorcluster)  [unwired: 11 in, 1 out]
            n109 = in-place {
              in-place-border: w254 -> [w262]
              in-place-border: w234 -> [w259]
              w263 = enum16{"Rising", "Falling"}."Falling"  # EdgeType
              w270 = i64 2500  # y
              w275 = 3.0  # Level(Voltage)
              w276 = SkidpadState."3lap"  # t
              n110 = in-place-cluster #7(w254) -> ("StateValue"=w277:T6, "CurrentRecordIndicator.LapProgress"=w274:T7)  [unwired: 4 out]
              n111 = Unbundle By Name(w262) -> ("FlagData.BlueFlag"=w261:picture, "InternalTimmer.2LapRefTime"=w260:i64)
              n112 = Tick Count (ms)() -> (millisecond timer value=w268:u32)
              n113 = To Quad Integer(1:w268) -> (0:w267:i64)
              n114 = call "DetectEdge(Analog).vi"("EdgeType"=w263, "Level(Voltage)"=w275, "Voltage"=w259) -> ("DetectedEdge"=w272:bool)  [unwired: 8 in]
              n115 = Subtract(x=w267, y=w260) -> (x-y=w266:i64)
              n116 = Greater?(x=w266, y=w270) -> (0:w269:bool)
              n117 = call "IntegerTimeToLabTime.vi"("inputTime(msec)"=w266) -> ("outputTime(mm-ss-sss)"=w265:string)  [unwired: 10 in]
              n118 = And(x=w269, y=w272) -> (x .and. y?=w271:bool)
              n119 = Bundle By Name(cluster=w274, "Lap-2"=w271) -> (w273:T7)
              n120 = Select(t=w276, s=w271, f=w277) -> (s? t:f=w264:T6)
              n121 = in-place-cluster #7("CurrentRecordIndicator.Flag"=w261, "InternalTimmer.2LapTime"=w266, "InternalTimmer.3LapRefTime"=w267, "StateValue"=w264, "CurrentRecordIndicator.Lab2"=w265, "CurrentRecordIndicator.LapProgress"=w273) -> (w237:T3)
            }
            n122 = Unbundle By Name(w237) -> ("EventProgressData"=w238:string[][], "CurrentRecordIndicator.CurrentEntry"=w245:string, "StateValue"=w239:T6)
            n123 = control-ref of="Attempt-1"() -> (w240:refnum<vi>)
            n124 = control-ref of="Attempt-2"() -> (w241:refnum<vi>)
            n125 = control-ref of="Attempt-3"() -> (w242:refnum<vi>)
            n126 = control-ref of="Attempt-4"() -> (w243:refnum<vi>)
            n127 = control-ref of="Lap-1"() -> (w246:refnum<vi>)
            n128 = control-ref of="Lap-2"() -> (w247:refnum<vi>)
            n129 = control-ref of="Lap-3"() -> (w248:refnum<vi>)
            n130 = control-ref of="Lap-4"() -> (w249:refnum<vi>)
            n131 = Build Array "Build Array"(w240, w241, w242, w243) -> (w244:refnum<vi>[])
            n132 = Build Array "Build Array"(w246, w247, w248, w249) -> (w250:refnum<vi>[])
            n133 = call "SkidpadLapLEDWinker.vi"("StateValue"=w239, "inputRefOfLED"=w250) -> ("outputError"=w235:errorcluster)  [unwired: 9 in]
            n134 = call "SkidpadAttemptLEDWinker.vi"("StateValue"=w239, "CurrentEntry"=w245, "EventProgressDataInput"=w238, "inputRefOfLED"=w244) -> ("outputError"=w236:errorcluster)  [unwired: 7 in]
            n135 = Merge Errors "Merge Errors"(w236, w235, w251, w252, w255) -> (w253:errorcluster)
          }
          frame "3lap" {
            n136 = call-poly <vilib>:"DAQmx Read.vi"("task/channels in"=w302, "error in"=w301) -> ("data"=w278:dbl, "error out"=w299:errorcluster)  [unwired: 11 in, 1 out]
            n137 = in-place {
              in-place-border: w298 -> [w309]
              in-place-border: w278 -> [w303]
              w306 = enum16{"Rising", "Falling"}."Falling"  # EdgeType
              w313 = i64 2500  # y
              w319 = 3.0  # Level(Voltage)
              w320 = SkidpadState."4lap"  # t
              n138 = in-place-cluster #8(w298) -> ("CurrentRecordIndicator.LapProgress"=w318:T7, "StateValue"=w305:T6)  [unwired: 3 out]
              n139 = Unbundle By Name(w309) -> ("FlagData.BlueFlag"=w308:picture, "InternalTimmer.3LapRefTime"=w307:i64)
              n140 = Tick Count (ms)() -> (millisecond timer value=w311:u32)
              n141 = To Quad Integer(1:w311) -> (0:w310:i64)
              n142 = call "DetectEdge(Analog).vi"("EdgeType"=w306, "Level(Voltage)"=w319, "Voltage"=w303) -> ("DetectedEdge"=w316:bool)  [unwired: 8 in]
              n143 = Subtract(x=w310, y=w307) -> (x-y=w314:i64)
              n144 = Greater?(x=w314, y=w313) -> (0:w312:bool)
              n145 = And(x=w312, y=w316) -> (x .and. y?=w315:bool)
              n146 = Select(t=w320, s=w315, f=w305) -> (s? t:f=w304:T6)
              n147 = Bundle By Name(cluster=w318, "Lap-3"=w315) -> (w317:T7)
              n148 = in-place-cluster #8("CurrentRecordIndicator.Flag"=w308, "InternalTimmer.3LapTime"=w314, "InternalTimmer.4LapRefTime"=w310, "CurrentRecordIndicator.LapProgress"=w317, "StateValue"=w304) -> (w281:T3)
            }
            n149 = Unbundle By Name(w281) -> ("EventProgressData"=w282:string[][], "CurrentRecordIndicator.CurrentEntry"=w289:string, "StateValue"=w283:T6)
            n150 = control-ref of="Attempt-1"() -> (w284:refnum<vi>)
            n151 = control-ref of="Attempt-2"() -> (w285:refnum<vi>)
            n152 = control-ref of="Attempt-3"() -> (w286:refnum<vi>)
            n153 = control-ref of="Attempt-4"() -> (w287:refnum<vi>)
            n154 = control-ref of="Lap-1"() -> (w290:refnum<vi>)
            n155 = control-ref of="Lap-2"() -> (w291:refnum<vi>)
            n156 = control-ref of="Lap-3"() -> (w292:refnum<vi>)
            n157 = control-ref of="Lap-4"() -> (w293:refnum<vi>)
            n158 = Build Array "Build Array"(w284, w285, w286, w287) -> (w288:refnum<vi>[])
            n159 = Build Array "Build Array"(w290, w291, w292, w293) -> (w294:refnum<vi>[])
            n160 = call "SkidpadLapLEDWinker.vi"("StateValue"=w283, "inputRefOfLED"=w294) -> ("outputError"=w279:errorcluster)  [unwired: 9 in]
            n161 = call "SkidpadAttemptLEDWinker.vi"("StateValue"=w283, "CurrentEntry"=w289, "EventProgressDataInput"=w282, "inputRefOfLED"=w288) -> ("outputError"=w280:errorcluster)  [unwired: 7 in]
            n162 = Merge Errors "Merge Errors"(w280, w279, w295, w296, w299) -> (w297:errorcluster)
          }
          frame "4lap" {
            n163 = call-poly <vilib>:"DAQmx Read.vi"("task/channels in"=w345, "error in"=w344) -> ("data"=w321:dbl, "error out"=w342:errorcluster)  [unwired: 11 in, 1 out]
            n164 = in-place {
              in-place-border: w341 -> [w351]
              in-place-border: w321 -> [w346]
              w347 = enum16{"Rising", "Falling"}."Falling"  # EdgeType
              w357 = i64 2500  # y
              w362 = 3.0  # Level(Voltage)
              w363 = SkidpadState."FinshRunning"  # t
              n165 = in-place-cluster #9(w341) -> ("StateValue"=w364:T6, "CurrentRecordIndicator.LapProgress"=w361:T7)  [unwired: 3 out]
              n166 = Unbundle By Name(w351) -> ("FlagData.BlueFlag"=w350:picture, "InternalTimmer.4LapRefTime"=w349:i64)
              n167 = Tick Count (ms)() -> (millisecond timer value=w355:u32)
              n168 = To Quad Integer(1:w355) -> (0:w354:i64)
              n169 = call "DetectEdge(Analog).vi"("EdgeType"=w347, "Level(Voltage)"=w362, "Voltage"=w346) -> ("DetectedEdge"=w359:bool)  [unwired: 8 in]
              n170 = Subtract(x=w354, y=w349) -> (x-y=w353:i64)
              n171 = Greater?(x=w353, y=w357) -> (0:w356:bool)
              n172 = call "IntegerTimeToLabTime.vi"("inputTime(msec)"=w353) -> ("outputTime(mm-ss-sss)"=w352:string)  [unwired: 10 in]
              n173 = And(x=w356, y=w359) -> (x .and. y?=w358:bool)
              n174 = Bundle By Name(cluster=w361, "Lap-4"=w358) -> (w360:T7)
              n175 = Select(t=w363, s=w358, f=w364) -> (s? t:f=w348:T6)
              n176 = in-place-cluster #9("CurrentRecordIndicator.Flag"=w350, "InternalTimmer.4LapTime"=w353, "StateValue"=w348, "CurrentRecordIndicator.Lab4"=w352, "CurrentRecordIndicator.LapProgress"=w360) -> (w324:T3)
            }
            n177 = Unbundle By Name(w324) -> ("EventProgressData"=w325:string[][], "CurrentRecordIndicator.CurrentEntry"=w332:string, "StateValue"=w326:T6)
            n178 = control-ref of="Attempt-1"() -> (w327:refnum<vi>)
            n179 = control-ref of="Attempt-2"() -> (w328:refnum<vi>)
            n180 = control-ref of="Attempt-3"() -> (w329:refnum<vi>)
            n181 = control-ref of="Attempt-4"() -> (w330:refnum<vi>)
            n182 = control-ref of="Lap-1"() -> (w333:refnum<vi>)
            n183 = control-ref of="Lap-2"() -> (w334:refnum<vi>)
            n184 = control-ref of="Lap-3"() -> (w335:refnum<vi>)
            n185 = control-ref of="Lap-4"() -> (w336:refnum<vi>)
            n186 = Build Array "Build Array"(w327, w328, w329, w330) -> (w331:refnum<vi>[])
            n187 = Build Array "Build Array"(w333, w334, w335, w336) -> (w337:refnum<vi>[])
            n188 = call "SkidpadLapLEDWinker.vi"("StateValue"=w326, "inputRefOfLED"=w337) -> ("outputError"=w322:errorcluster)  [unwired: 9 in]
            n189 = call "SkidpadAttemptLEDWinker.vi"("StateValue"=w326, "CurrentEntry"=w332, "EventProgressDataInput"=w325, "inputRefOfLED"=w331) -> ("outputError"=w323:errorcluster)  [unwired: 7 in]
            n190 = Merge Errors "Merge Errors"(w323, w322, w338, w339, w342) -> (w340:errorcluster)
          }
          frame "FinshRunning" {
            w365 = FALSE
            n191 = in-place {
              in-place-border: w366 -> [w373]
              w378 = SkidpadState."LogRecord"  # State
              w379 = "Finsh Line"  # CurrentRecordIndicator.CurrentState
              n192 = in-place-cluster #10(w366) -> ("InternalTimmer.2LapTime"=w376:i64, "InternalTimmer.4LapTime"=w375:i64)  [unwired: 5 out]
              n193 = Unbundle By Name(w373) -> ("FlagData.CheckFlag"=w372:picture)
              n194 = Add(x=w376, y=w375) -> (x+y=w374:i64)
              n195 = call "IntegerTimeToLabTime.vi"("inputTime(msec)"=w374) -> ("outputTime(mm-ss-sss)"=w377:string)  [unwired: 10 in]
              n196 = in-place-cluster #10("CurrentRecordIndicator.Flag"=w372, "CurrentRecordIndicator.Message"=w379, "InternalTimmer.2LapTime"=w376, "InternalTimmer.4LapTime"=w375, "InternalTimmer.TotalLabTime"=w374, "CurrentRecordIndicator.TotalLabTime"=w377, "StateValue"=w378) -> (w371:T3)
            }
            n197 = Merge Errors "Merge Errors"(w369, w368, w367) -> (w370:errorcluster)
            n198 = local write "Ready"(w365) -> ()
          }
          frame "LogRecord" {
            w384 = "LoggingData"  # SubFolderName
            w392 = TRUE  # append to file? (F)
            w402 = 0.0  # data
            n199 = Unbundle By Name(w380) -> ("CurrentRecordIndicator.CurrentEntry"=w382:string, "CurrentRecordIndicator.CurrentSchool"=w409:string, "CurrentRecordIndicator.Lab2"=w408:string, "CurrentRecordIndicator.Lab4"=w407:string, "CurrentRecordIndicator.TotalLabTime"=w406:string, "InternalTimmer.TotalLabTime"=w386:i64)
            n200 = call-poly <vilib>:"DAQmx Write.vi"("task/channels in"=w401, "data"=w402, "error in"=w399) -> ("task out"=w404:refnum<k21>, "error out"=w403:errorcluster)  [unwired: 10 in, 1 out]
            n201 = call <vilib>:"DAQmx Stop Task.vi"("task/channels in"=w404, "error in"=w403) -> ("error out"=w396:errorcluster)  [unwired: 12 in, 1 out]
            n202 = call <vilib>:"DAQmx Stop Task.vi"("task/channels in"=w400, "error in"=w398) -> ("error out"=w395:errorcluster)  [unwired: 12 in, 1 out]
            n203 = Current VI's Path() -> (path=w383:path)
            n204 = call "ScreenShotFrontPannel.vi"("SubFolderName"=w384, "FileName"=w382, "vi path"=w383) -> ("error out"=w381:errorcluster)  [unwired: 8 in]
            n205 = Number To Decimal String(number=w386) -> (decimal integer string=w405:string)  [unwired: 1 in]
            n206 = Build Array "Build Array"(w382, w409, w408, w407, w406, w405) -> (w393:string[])
            n207 = call-poly <vilib>:"Write Delimited Spreadsheet.vi"("file path (dialog if empty)"=w394, "1D data"=w393, "append to file? (new file:F)"=w392) -> ("new file path (Not A Path if cancelled)"=w391:path, "error out"=w390:errorcluster)  [unwired: 11 in]
            n208 = in-place {
              in-place-border: w391 -> [w432]
              in-place-border: w390 -> [w431]
              in-place-border: w389 -> [w430]
              in-place-border: [w428] -> w385
              in-place-border: w380 -> [w426]
              w417 = 5  # IndexColumn
              w418 = 4  # Index
              w419 = 1  # Index
              w420 = 0  # Index
              w429 = SkidpadState."HardwareRelease"  # StateValue
              n209 = in-place-cluster #11(w380) -> ("EventProgressData"=w433:string[][])  [unwired: 5 out]
              n210 = Unbundle By Name(w426) -> ("CurrentRecordIndicator.CurrentEntry"=w422:string)
              n211 = call-poly <vilib>:"Read Delimited Spreadsheet.vi"("file path (dialog if empty)"=w432, "error in (no error)"=w431) -> ("new file path (Not A Path if cancelled)"=w416:path, "all rows"=w427:string[][], "error out"=w415:errorcluster)  [unwired: 8 in, 3 out]
              n212 = call "RecordDataToEventProgressData.vi"("RecordData"=w427, "inputEventProgressData"=w433) -> ("outputEventProgressData"=w425:string[][])  [unwired: 9 in]
              n213 = call "ReadBestRecord.vi"("IndexColumn"=w417, "ErrorInput"=w415, "FilepathInput"=w416) -> ("ErrorOutput"=w414:errorcluster, "Data"=w421:string[])  [unwired: 6 in, 1 out]
              n214 = call "EventProgressToEventCount.vi"("CurrentEntry"=w422, "EventProgressDataInput"=w425) -> ("EventCount"=w424:i32)  [unwired: 9 in]
              n215 = call "EventCounterToEventCounterCluster.vi"("EventCount"=w424) -> ("CurrentRecordIndicator.EventCount"=w423:T9)  [unwired: 10 in]
              n216 = Index Array "Index Array"(array=w421, index #1=w420, index #2=w419, index #3=w418) -> (element #1=w413:string, element #2=w412:string, element #3=w411:string)
              n217 = in-place-cluster #11("StateValue"=w429, "EventProgressData"=w425, "CurrentRecordIndicator.EventCount"=w423, "BestRecordIndicator.BestEntry"=w413, "BestRecordIndicator.BestUniv"=w412, "BestRecordIndicator.BestTime"=w411) -> (w388:T3)
              n218 = Merge Errors "Merge Errors"(w430, w414) -> (w428:errorcluster)
            }
            n219 = Unbundle By Name(w388) -> ("EventProgressData"=w387:string[][])
            n220 = Merge Errors "Merge Errors"(w385, w381, w396, w395) -> (w397:errorcluster)
            n221 = local write "Progress"(w387) -> ()
          }
          frame "HardwareRelease" {
            w434 = 0.0  # data
            n222 = in-place {
              w448 = SkidpadState."WaittingforNext"  # StateValue
              n223 = in-place-cluster #12(w447) -> ()  [unwired: 1 out]
              n224 = in-place-cluster #12("StateValue"=w448) -> (w435:T3)
            }
            n225 = call-poly <vilib>:"DAQmx Write.vi"("task/channels in"=w446, "data"=w434, "error in"=w445) -> ("task out"=w444:refnum<k21>, "error out"=w443:errorcluster)  [unwired: 10 in, 1 out]
            n226 = call <vilib>:"DAQmx Stop Task.vi"("task/channels in"=w444, "error in"=w443) -> ("error out"=w439:errorcluster)  [unwired: 12 in, 1 out]
            n227 = call <vilib>:"DAQmx Stop Task.vi"("task/channels in"=w442, "error in"=w441) -> ("error out"=w440:errorcluster)  [unwired: 12 in, 1 out]
            n228 = Merge Errors "Merge Errors"(w438, w439, w440) -> (w437:errorcluster)
          }
          frame "WaittingforNext" {
            n229 = Merge Errors "Merge Errors"(w450, w452, w451) -> (w453:errorcluster)
            n230 = in-place {
              in-place-border: w449 -> [w457]
              w460 = SkidpadState."Initial"  # State
              n231 = in-place-cluster #13(w449) -> ("StateValue"=w458:T6)
              n232 = Unbundle By Name(w457) -> ("NextEntry"=w456:bool)
              n233 = Select(t=w460, s=w456, f=w458) -> (s? t:f=w459:T6)
              n234 = in-place-cluster #13("StateValue"=w459) -> (w454:T3)
            }
          }
          frame "ProgramStop" {
            w480 = FALSE  # Ready
            n235 = call <vilib>:"DAQmx Clear Task.vi"("task in"=w485, "error in"=w481) -> ("error out"=w483:errorcluster)  [unwired: 13 in]
            n236 = call <vilib>:"DAQmx Clear Task.vi"("task in"=w487, "error in"=w482) -> ("error out"=w486:errorcluster)  [unwired: 13 in]
            n237 = in-place {
              in-place-border: w478 -> [w489]
              w490 = "Halted Program"  # CurrentRecordIndicator.CurrentState
              n238 = in-place-cluster #14(w478) -> ()  [unwired: 2 out]
              n239 = Unbundle By Name(w489) -> ("FlagData.RedFlag"=w488:picture)
              n240 = in-place-cluster #14("CurrentRecordIndicator.Flag"=w488, "CurrentRecordIndicator.Message"=w490) -> (w463:T3)
            }
            n241 = Unbundle By Name(w463) -> ("EventProgressData"=w465:string[][], "CurrentRecordIndicator.CurrentEntry"=w471:string, "StateValue"=w464:T6)
            n242 = control-ref of="Attempt-1"() -> (w466:refnum<vi>)
            n243 = control-ref of="Attempt-2"() -> (w467:refnum<vi>)
            n244 = control-ref of="Attempt-3"() -> (w468:refnum<vi>)
            n245 = control-ref of="Attempt-4"() -> (w469:refnum<vi>)
            n246 = control-ref of="Lap-1"() -> (w472:refnum<vi>)
            n247 = control-ref of="Lap-2"() -> (w473:refnum<vi>)
            n248 = control-ref of="Lap-3"() -> (w474:refnum<vi>)
            n249 = control-ref of="Lap-4"() -> (w475:refnum<vi>)
            n250 = Build Array "Build Array"(w472, w473, w474, w475) -> (w476:refnum<vi>[])
            n251 = Build Array "Build Array"(w466, w467, w468, w469) -> (w470:refnum<vi>[])
            n252 = call "SkidpadLapLEDWinker.vi"("StateValue"=w464, "inputRefOfLED"=w476) -> ("outputError"=w462:errorcluster)  [unwired: 9 in]
            n253 = call "SkidpadAttemptLEDWinker.vi"("StateValue"=w464, "CurrentEntry"=w471, "EventProgressDataInput"=w465, "inputRefOfLED"=w470) -> ("outputError"=w461:errorcluster)  [unwired: 7 in]
            n254 = local write "Ready"(w480) -> ()
            n255 = Merge Errors "Merge Errors"(w461, w462, w477, w483, w486) -> (w484:errorcluster)
          }
        }
        n256 = Unbundle By Name(w61) -> ("ProgramStop"=w63:bool)
        n257 = in-place {
          in-place-border: w58 -> [w494]
          in-place-border: w63 -> [w493]
          in-place-border: w57 -> [w491]
          n258 = in-place-cluster #15(w61) -> ("StateValue"=w492:T6)
          n259 = Or(x=w493, y=w494) -> (x .or. y?=w495:bool)
          n260 = Select(t=w491, s=w495, f=w492) -> (s? t:f=w496:T6)
          n261 = in-place-cluster #15("StateValue"=w496) -> (w73:T3)
        }
        n262 = Unbundle By Name(w73) -> ("CurrentRecordIndicator"=→"CurrentRecordIndicator":T1, "BestRecordIndicator"=→"BestRecordIndicator":T2)
        n263 = Wait Until Next ms Multiple(millisecond multiple=w66) -> ()  [unwired: 1 out]
      }
    }
    frame #2 {
      n264 = call <vilib>:"Simple Error Handler.vi"("error in (no error)"=w497) -> ()  [unwired: 4 in, 5 out]
    }
  }
